vi "PostSub Steps LV PPS.vi"(9 "Socket Index":i16, 10 "PPS Config In":T1={"VISA Resource"="", "Voltage Level (0.0 V)"=0.0, "CURRent Limit (0.0 A)"=0.0, "OVP LEVEL (0V)"=0.0, "Enable OVP (T: Enable)"=TRUE, "OCP LEVEL (0A)"=0.0, "Enable OCP (T: Enable)"=TRUE, "Value Out"="", "Value In"="", "Actual Voltage Level (V)"=0.0, "Actual Current Limit (A)"=0.0, "Select Instrument"="", "Enable Output"=FALSE, "PPS Operation"=enum."Close", "Type"=0} {"Type" items=["Voltage", "Current"]; "Actual Current Limit (A)" format="%.2f"; "Actual Voltage Level (V)" format="%.2f"; "OCP LEVEL (0A)" format="%.2f"; "OVP LEVEL (0V)" format="%.2f"; "Voltage Level (0.0 V)" format="%.2f"}, 11 "Sequence Context In":refnum<k7>) -> (0 "error out":errorcluster, 2 "PPS Config Out":T1={"VISA Resource"="", "Voltage Level (0.0 V)"=0.0, "CURRent Limit (0.0 A)"=0.0, "OVP LEVEL (0V)"=0.0, "Enable OVP (T: Enable)"=TRUE, "OCP LEVEL (0A)"=0.0, "Enable OCP (T: Enable)"=TRUE, "Value Out"="", "Value In"="", "Actual Voltage Level (V)"=0.0, "Actual Current Limit (A)"=0.0, "Select Instrument"="", "Enable Output"=FALSE, "PPS Operation"=enum."Close", "Type"=0} {"Type" items=["Voltage", "Current"]; "Actual Current Limit (A)" format="%.2f"; "Actual Voltage Level (V)" format="%.2f"; "OCP LEVEL (0A)" format="%.2f"; "OVP LEVEL (0V)" format="%.2f"; "Voltage Level (0.0 V)" format="%.2f"}, 3 "Report Text":string)   [LabVIEW 2023, in "LTT_TeststandSteptypes.lvlib"]
uses:
  LTT_TeststandSteptypes.lvlib
  HardwareAbstractionLayer_LVOOP/PowerSupply/Teststand/Control/PPS StepType Control.ctl
  HardwareAbstractionLayer_LVOOP/PowerSupply/Control/PPS Configure Data.ctl
  HardwareAbstractionLayer_LVOOP/PowerSupply/IT-M3904D/IT-M3904D.lvclass
  D:/eDCU LTT/VT LTT Project/Source Code/HardwareAbstractionLayer_LVOOP/PowerSupply/PowerSupply.lvclass
  <vilib>/addons/TestStand/_TSUtility.llb/TestStand - Set Property Value (Number).vi
  HardwareAbstractionLayer_LVOOP/PowerSupply/PowerSupply.lvclass
  HardwareAbstractionLayer_LVOOP/PowerSupply/IT-M6018C/IT-M6018C.lvclass
  HardwareAbstractionLayer_LVOOP/Database/Database.lvclass
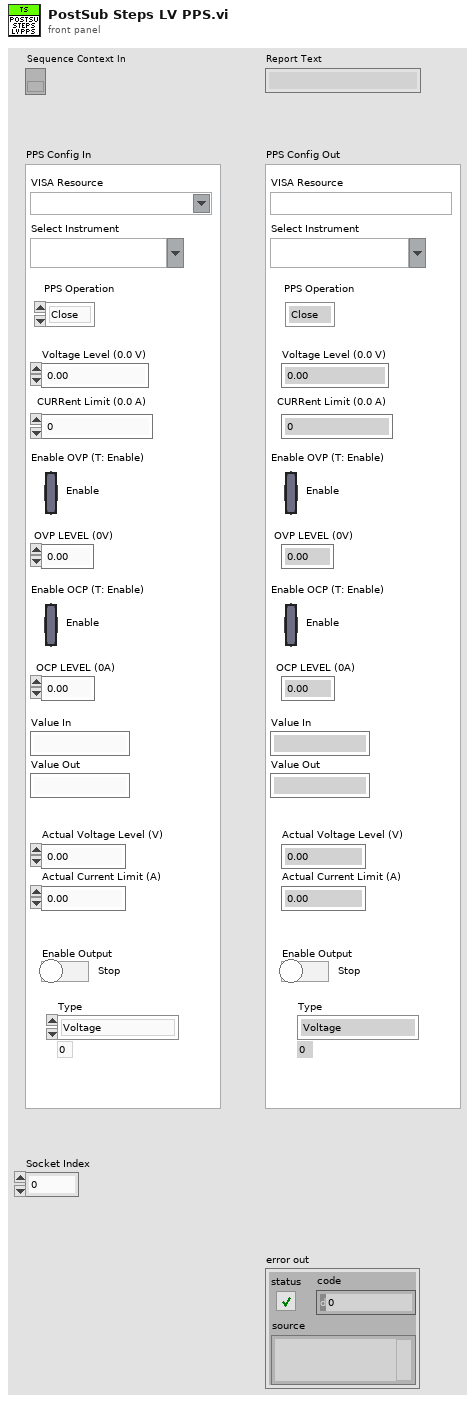
[diagram p1: front panel]
types:
  T1 = typedef "HardwareAbstractionLayer_LVOOP.lvlib/PowerSupply.lvclass/PPS StepType Control.ctl" = cluster{"VISA Resource":refnum<visa-resource-name>, "Voltage Level (0.0 V)":dbl, "CURRent Limit (0.0 A)":dbl, "OVP LEVEL (0V)":dbl, "Enable OVP (T: Enable)":bool, "OCP LEVEL (0A)":dbl, "Enable OCP (T: Enable)":bool, "Value Out":string, "Value In":string, "Actual Voltage Level (V)":dbl, "Actual Current Limit (A)":dbl, "Select Instrument":string, "Enable Output":bool, "PPS Operation":enum32{"Init", "Self Test", "Configure", "Measure", "Close"}, "Type":u16}
  T2 = enum32{"Init", "Self Test", "Configure", "Measure", "Close"}
  T3 = typedef "HardwareAbstractionLayer_LVOOP.lvlib/PowerSupply.lvclass/PPS Configure Data.ctl" = cluster{"Voltage Level (0.0 V)":dbl, "CURRent Limit (0.0 A)":dbl, "OVP LEVEL (0V)":dbl, "OCP LEVEL (0A)":dbl, "Enable OVP (T: Enable)":bool, "Enable OCP (T: Enable)":bool, "Enable Output ":bool, "Delays OCP":dbl, "Delays OVP":dbl, "Mode(0:Voltage)":u16, "CURRent Level (0.0 A)":dbl, "Voltage Limit (0.0 V)":dbl}
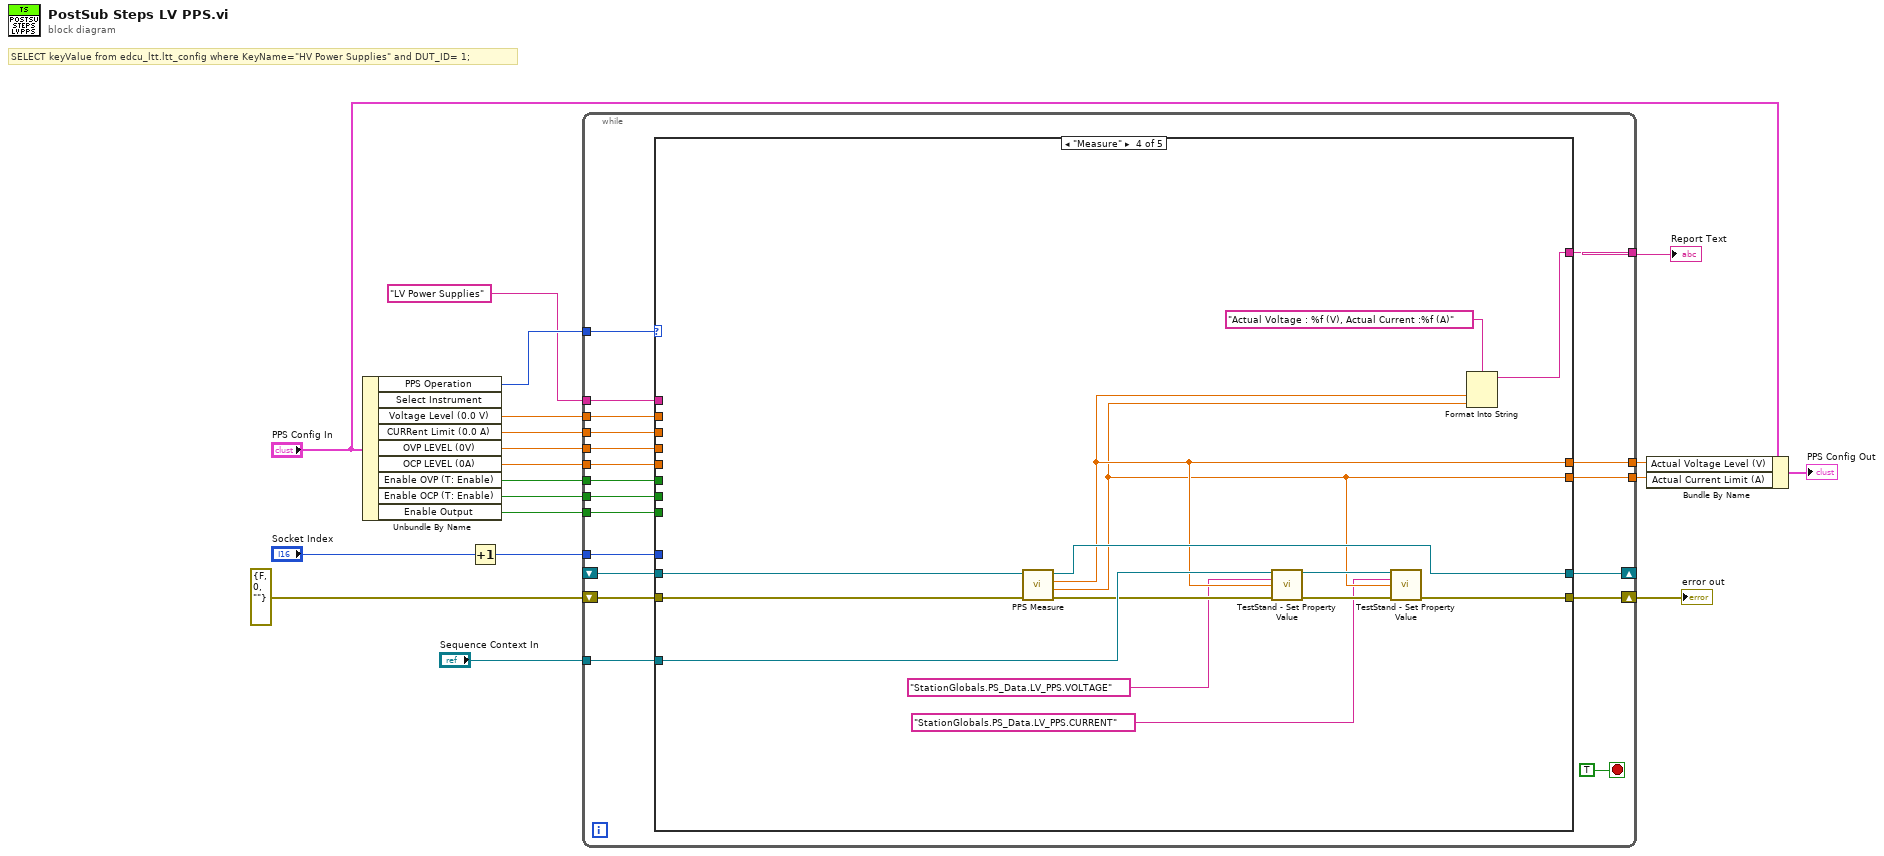
[diagram p0: block diagram]
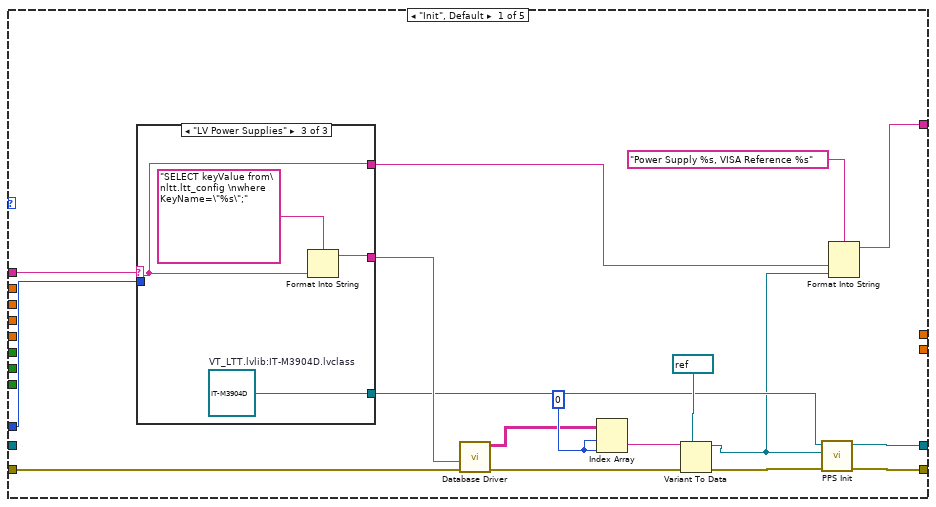
[diagram p2: hidden frame]
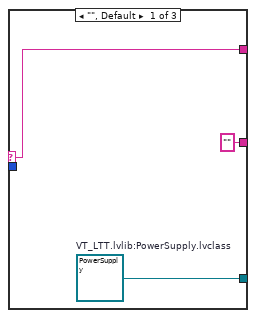
[diagram p3: hidden frame]
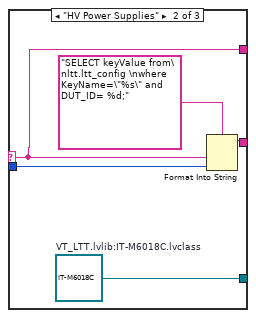
[diagram p4: hidden frame]
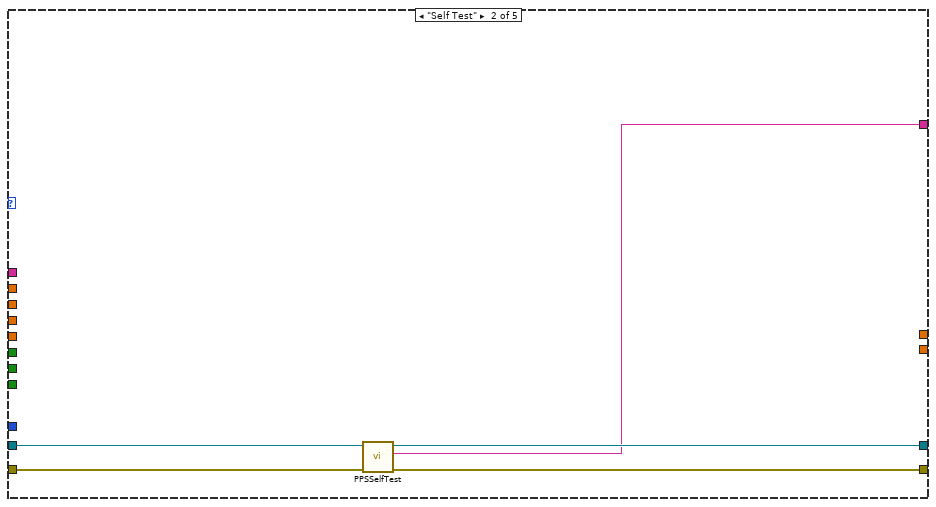
[diagram p5: hidden frame]
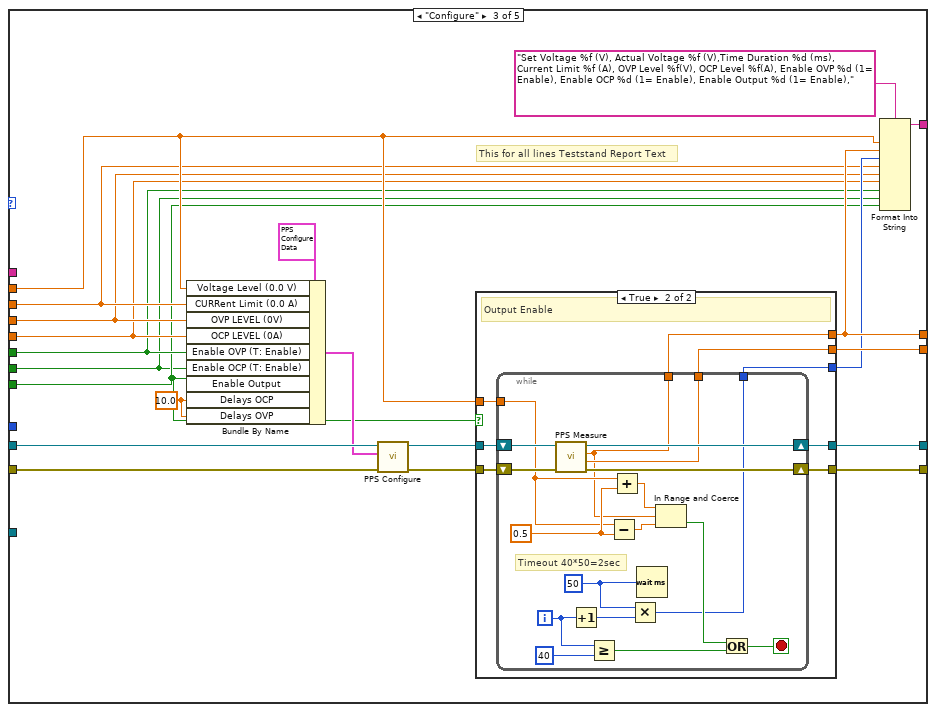
[diagram p6: hidden frame]
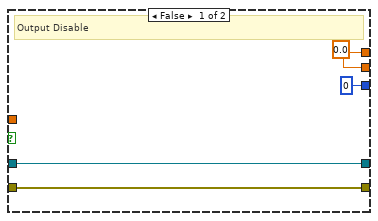
[diagram p7: hidden frame]
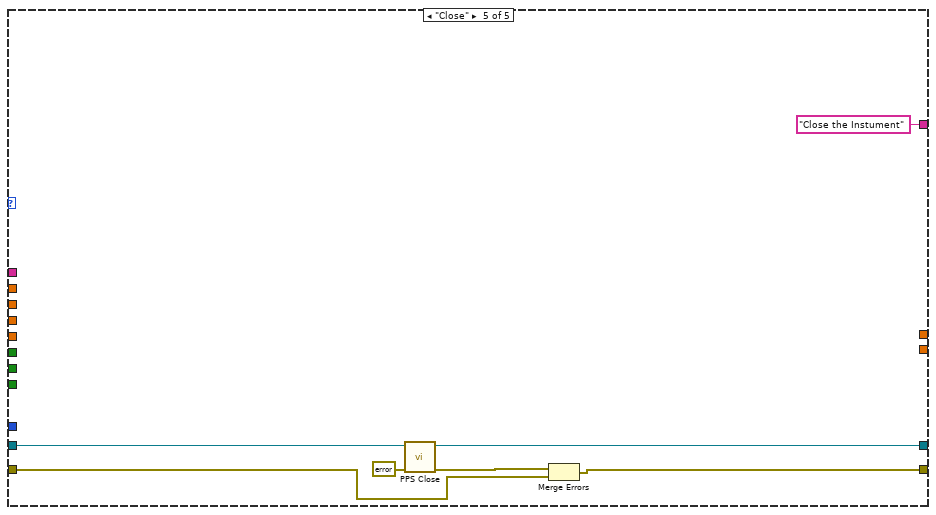
[diagram p8: hidden frame]
diagram:
  # "SELECT keyValue from edcu_ltt.ltt_config where KeyName=\"HV Power Supplies\" and DUT_ID= 1;"
  n1 = Unbundle By Name("PPS Config In") -> ("PPS Operation"=w19:T2, "Voltage Level (0.0 V)"=w16:dbl, "CURRent Limit (0.0 A)"=w15:dbl, "OVP LEVEL (0V)"=w14:dbl, "OCP LEVEL (0A)"=w13:dbl, "Enable OVP (T: Enable)"=w12:bool, "Enable OCP (T: Enable)"=w11:bool, "Enable Output"=w10:bool)  [unwired: 1 out]
  n2 = Increment(x="Socket Index") -> (x+1=w3:i16)
  n3 = while {
    tunnel: w19 -> [w37]
    tunnel: "LV Power Supplies" ("Select Instrument") -> [w36]
    shift-right: [w33] -> _
    shift-left: _ -> [w32]
    shift-right: [w34] -> w17
    shift-left: errorcluster {"status"=FALSE, "code"=0, "source"=""} ("error in") -> [w35]
    tunnel: w16 -> [w31]
    tunnel: w15 -> [w30]
    tunnel: w14 -> [w29]
    tunnel: w13 -> [w28]
    tunnel: w12 -> [w27]
    tunnel: w11 -> [w26]
    tunnel: w10 -> [w25]
    tunnel: w3 -> [w24]
    tunnel: [w23] -> w8
    tunnel: [w22] -> w5
    tunnel: [w21] -> w4
    tunnel: "Sequence Context In" -> [w20]
    stop <- TRUE stop-if-true
    n4 = case shown="\"Measure\"" w37 {
      tunnel: w36 -> [w55 _ _ _ _]
      tunnel: w35 -> [w45 w71 w92 w131 w138]
      tunnel: [w54 w70 w89 w128 w139] -> w34
      tunnel: [w53 w69 w88 w136 w142] -> w33
      tunnel: w32 -> [_ w72 w93 w137 w143]
      tunnel: w31 -> [_ _ w85 _ _]
      tunnel: w30 -> [_ _ w79 _ _]
      tunnel: w29 -> [_ _ w78 _ _]
      tunnel: w28 -> [_ _ w77 _ _]
      tunnel: w27 -> [_ _ w76 _ _]
      tunnel: w26 -> [_ _ w74 _ _]
      tunnel: w25 -> [_ _ w75 _ _]
      tunnel: w24 -> [w52 _ _ _ _]
      tunnel: [w42 w68 w84 w135 "Close the Instument" ("Self-Test Result Message")] -> w23
      tunnel: [_ _ w83 w127 _] -> w22
      tunnel: [_ _ w82 w126 _] -> w21
      tunnel: w20 -> [_ _ _ w133 _]
      frame "Init", Default {
        w51 = 0 ("index (row)")
        n5 = case shown="\"LV Power Supplies\"" w55 {
          selector: w55 -> [w56 w59 w64]
          tunnel: [w58 w63 w67] -> w43
          tunnel: w52 -> [_ w61 _]
          tunnel: ["" w60 w65] -> w47
          tunnel: [w56 w59 w64] -> w40
          frame "", Default {
            w58 = refnum<class "PowerSupply.lvclass"> refnum  # VT_LTT.lvlib:PowerSupply.lvclass
          }
          frame "HV Power Supplies" {
            w63 = refnum<class "IT-M6018C.lvclass"> refnum  # VT_LTT.lvlib:IT-M6018C.lvclass
            n6 = Format Into String(format string="SELECT keyValue from\nltt.ltt_config \nwhere KeyName=\"%s\" and DUT_ID= %d;", w59, w61) -> (resulting string=w60:string)  [unwired: 2 in, 1 out]
          }
          frame "LV Power Supplies" {
            w67 = refnum<class "IT-M3904D.lvclass"> refnum  # VT_LTT.lvlib:IT-M3904D.lvclass
            n7 = Format Into String(format string="SELECT keyValue from\nltt.ltt_config \nwhere KeyName=\"%s\";", w64) -> (resulting string=w65:string)  [unwired: 2 in, 1 out]
          }
        }
        n8 = call "Database Driver.vi"("error in"=w45, "SQL query"=w47) -> ("error out"=w44:errorcluster, "data"=w46:string[][])  [unwired: 6 in, 2 out]
        n9 = Index Array(array=w46, index (row)=w51, index (col)=w51) -> (element=w48:string)
        n10 = Variant To Data(error in=w44, type=refnum<visa-resource-name> "LV" ("VISA resource name"), Variant=w48) -> (data=w39:refnum<visa-resource-name>, error out=w50:errorcluster)
        n11 = call-dynamic "PPS Init.vi"("error in (no error)"=w50, "VISA resource name"=w39, "PowerSupply in"=w43) -> ("error out"=w54:errorcluster, "PowerSupply out"=w53:refnum<class "PowerSupply.lvclass">)  [unwired: 7 in]
        n12 = Format Into String(format string="Power Supply %s, VISA Reference %s", w40, w39) -> (resulting string=w42:string)  [unwired: 2 in, 1 out]
      }
      frame "Self Test" {
        n13 = call-dynamic "PPSSelfTest.vi"("error in (no error)"=w71, "PowerSupply in"=w72) -> ("error out"=w70:errorcluster, "Self-Test Result Message"=w68:string, "PowerSupply out"=w69:refnum<class "PowerSupply.lvclass">)  [unwired: 7 in]
      }
      frame "Configure" {
        w73 = 10.0 ("Delays OCP")
        # "This for all lines Teststand Report Text"
        n14 = Bundle By Name(cluster=T3 {"Voltage Level (0.0 V)"=0.0, "CURRent Limit (0.0 A)"=0.0, "OVP LEVEL (0V)"=0.0, "OCP LEVEL (0A)"=0.0, "Enable OVP (T: Enable)"=TRUE, "Enable OCP (T: Enable)"=TRUE, "Enable Output "=TRUE, "Delays OCP"=0.0, "Delays OVP"=0.0, "Mode(0:Voltage)"=0, "CURRent Level (0.0 A)"=0.0, "Voltage Limit (0.0 V)"=0.0} ("Configure"), "Voltage Level (0.0 V)"=w85, "CURRent Limit (0.0 A)"=w79, "OVP LEVEL (0V)"=w78, "OCP LEVEL (0A)"=w77, "Enable OVP (T: Enable)"=w76, "Enable OCP (T: Enable)"=w74, "Enable Output"=w75, "Delays OCP"=w73, "Delays OVP"=w73) -> (w90:T3)
        n15 = call-dynamic "PPS Configure.vi"("error in (no error)"=w92, "Configure"=w90, "PowerSupply in"=w93) -> ("error out"=w81:errorcluster, "PowerSupply out"=w87:refnum<class "PowerSupply.lvclass">)  [unwired: 7 in]
        n16 = case shown="True" w75 {
          tunnel: w81 -> [w96 w105]
          tunnel: [w96 w104] -> w89
          tunnel: [w97 w103] -> w88
          tunnel: w87 -> [w97 w102]
          tunnel: w85 -> [_ w99]
          tunnel: [w95 w101] -> w83
          tunnel: [w95 w100] -> w82
          tunnel: [u32 0 w98] -> w80
          frame False {
            w95 = 0.0 ("Actual Voltage Level (V)")
            # "Output Disable"
          }
          frame True {
            # "Output Enable"
            n17 = while {
              tunnel: [w111] -> w101
              tunnel: [w119] -> w100
              shift-right: [w122] -> w104
              shift-left: w105 -> [w123]
              shift-right: [w121] -> w103
              shift-left: w102 -> [w120]
              tunnel: w99 -> [w112]
              tunnel: [w109] -> w98
              i -> [w108]
              stop <- w116 stop-if-true
              w114 = 0.5
              w110 = u32 50 ("milliseconds to wait")
              # "Timeout 40*50=2sec"
              n18 = call-dynamic "PPS Measure.vi"("error in (no error)"=w123, "PowerSupply in"=w120) -> ("error out"=w122:errorcluster, "Actual Current Limit (A)"=w119:dbl, "Actual Voltage Level (V)"=w111:dbl, "PowerSupply out"=w121:refnum<class "PowerSupply.lvclass">)  [unwired: 6 in]
              n19 = Increment(x=w108) -> (x+1=w106:i32)
              n20 = Greater Or Equal?(x=w108, y=40) -> (x >= y?=w118:bool)
              n21 = Subtract(x=w112, y=w114) -> (x-y=w113:dbl)
              n22 = Add(x=w112, y=w114) -> (x+y=w115:dbl)
              n23 = Multiply(x=w110, y=w106) -> (x*y=w109:u32)
              n24 = Wait (ms)(milliseconds to wait=w110) -> ()  [unwired: 1 out]
              n25 = In Range and Coerce(upper limit=w115, x=w111, lower limit=w113) -> (In Range?=w117:bool)  [unwired: 1 out]
              n26 = Or(x=w117, y=w118) -> (x .or. y?=w116:bool)
            }
          }
        }
        n27 = Format Into String(format string="Set Voltage %f (V), Actual Voltage %f (V),Time Duration %d (ms), Current Limit %f (A), OVP Level %f(V), OCP Level %f(A), Enable OVP %d (1= Enable), Enable OCP %d (1= Enable), Enable Output %d (1= Enable),", w85, w83, w80, w79, w78, w77, w76, w74, w75) -> (resulting string=w84:string)  [unwired: 2 in, 1 out]
      }
      frame "Measure" {
        n28 = call-dynamic "PPS Measure.vi"("error in (no error)"=w131, "PowerSupply in"=w137) -> ("error out"=w130:errorcluster, "Actual Current Limit (A)"=w126:dbl, "Actual Voltage Level (V)"=w127:dbl, "PowerSupply out"=w136:refnum<class "PowerSupply.lvclass">)  [unwired: 6 in]
        n29 = call-poly <vilib>:"TestStand - Set Property Value.vi"("Sequence Context In"=w133, "Lookup String"="StationGlobals.PS_Data.LV_PPS.VOLTAGE", "New Value"=w127, "error in (no error)"=w130) -> ("Sequence Context Out"=w132:refnum<k7>, "error out"=w129:errorcluster)  [unwired: 10 in]
        n30 = call-poly <vilib>:"TestStand - Set Property Value.vi"("Sequence Context In"=w132, "Lookup String"="StationGlobals.PS_Data.LV_PPS.CURRENT", "New Value"=w126, "error in (no error)"=w129) -> ("error out"=w128:errorcluster)  [unwired: 10 in, 1 out]
        n31 = Format Into String(format string="Actual Voltage : %f (V), Actual Current :%f (A)", w127, w126) -> (resulting string=w135:string)  [unwired: 2 in, 1 out]
      }
      frame "Close" {
        n32 = call-dynamic "PPS Close.vi"("error in (no error)"=errorcluster {"status"=FALSE, "code"=0, "source"=""}, "PowerSupply in"=w143) -> ("error out"=w144:errorcluster, "PowerSupply out"=w142:refnum<class "PowerSupply.lvclass">)  [unwired: 8 in]
        n33 = Merge Errors(w144, w138) -> (w139:errorcluster)
      }
    }
  }
  "error out" <- w17
  "Report Text" <- w8
  n34 = Bundle By Name(cluster="PPS Config In", "Actual Voltage Level (V)"=w5, "Actual Current Limit (A)"=w4) -> (→"PPS Config Out":T1)
